vi "Laboratory_practice12.vi"() -> ()   [LabVIEW 2021]
uses:
  <vilib>/Waveform/WDTFileIO.llb/Export Waveforms To Spreadsheet File (1D).vi
panel:
  out "Waveform 1 Graph":dynamicdata(graph)
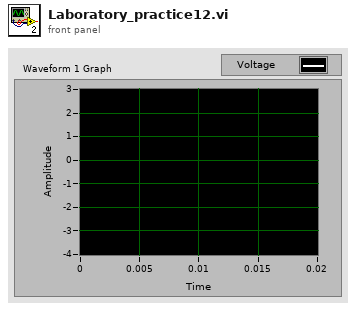
[diagram p1: front panel]
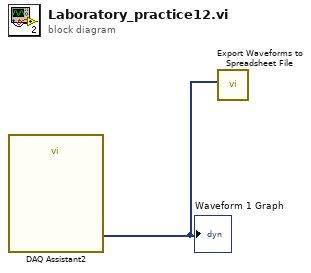
[diagram p0: block diagram]
diagram:
  n1 = call "DAQ Assistant2"() -> ("data"=w1:dynamicdata)  [unwired: 17 in, 2 out]
  "Waveform 1 Graph" <- w1
  n2 = call-poly <vilib>:"Export Waveforms to Spreadsheet File.vi"("waveforms"=w1) -> ()  [unwired: 9 in, 2 out]
